vi "GetSweepData.vi"(8 "error in (no error)":errorcluster, 10 "Current Channel":string, 11 "map":T1) -> (0 "error out":errorcluster, 3 "DataSet":T2)   [LabVIEW 2017, in "EmsaTestPanel.lvlib"]
uses:
  <vilib>/addons/InsightCM/Devices/Shared/Emsa/EmsaTestPanel/EmsaTestPanel.lvlib
  <vilib>/addons/InsightCM/MessageBus/Base/controls/DataSetByteData.ctl
  <vilib>/addons/InsightCM/MessageBus/Base/controls/KeyValuePair.ctl
  <vilib>/addons/PointValueMap/controls/PointMap.ctl
  <vilib>/addons/InsightCM/Utilities/PropertyHelpers/PropertyHelpers.lvlib
  <vilib>/addons/InsightCM/Devices/Shared/Emsa/EmsaAcquisition/EmsaAcquisition.lvlib
  <vilib>/addons/InsightCM/Devices/Shared/Emsa/EmsaDataEventCreator/EmsaDataEventCreator.lvlib
  <vilib>/addons/PointValueMap/PointValueMap.lvlib
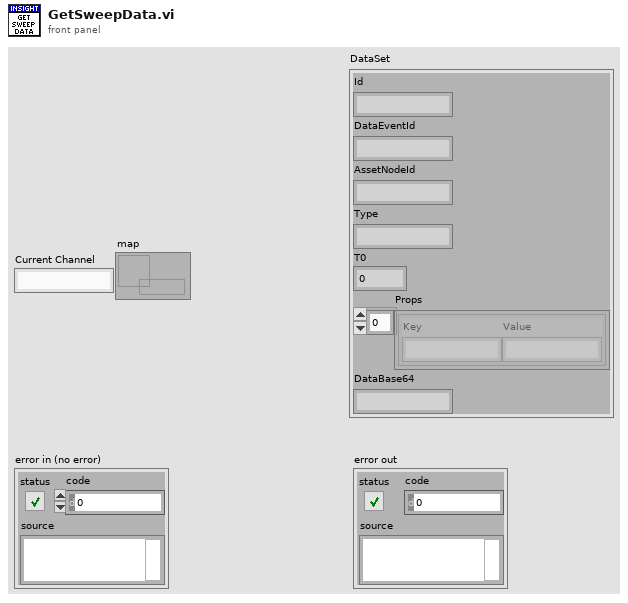
[diagram p1: front panel]
types:
  T1 = typedef "PointValueMap.lvlib/PointMap.ctl" = refnum<data-value>
  T2 = typedef "DataSetByteData.ctl" = cluster{"Id":string, "DataEventId":string, "AssetNodeId":string, "Type":string, "T0":i64, "Props":T3[], "DataBase64":string}
  T3 = typedef "KeyValuePair.ctl" = cluster{"Key":string, "Value":string}
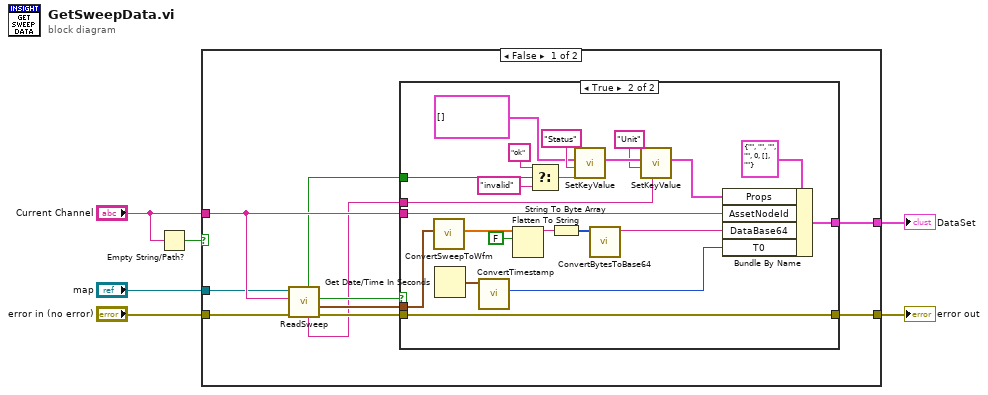
[diagram p0: block diagram]
diagram:
  n1 = Empty String/Path?(string/path="Current Channel") -> (empty?=w5:bool)
  n2 = case shown="False" w5 {
    tunnel: [w16 w40] -> w3
    tunnel: "error in (no error)" -> [w12 w40]
    tunnel: "Current Channel" -> [w14 _]
    tunnel: [w15 _] -> w2
    tunnel: "map" -> [w9 _]
    frame False {
      n3 = call <vilib>:"ReadSweep.vi"("error in (no error)"=w12, "channel"=w14, "map"=w9) -> ("error out"=w11:errorcluster, "sweep"=w10:cluster{"frequency":dbl, "amplitude":dbl}[], "found"=w13:bool, "unit"=w7:string, "valid"=w8:bool)  [unwired: 3 in, 1 out]
      n4 = case shown="True" w13 {
        tunnel: [w17 w35] -> w16
        tunnel: w11 -> [w17 w35]
        tunnel: w10 -> [_ w34]
        tunnel: w14 -> [_ w39]
        tunnel: [_ w37] -> w15
        tunnel: w8 -> [_ w30]
        tunnel: w7 -> [_ w18]
        frame False {
        }
        frame True {
          n5 = call <vilib>:"ConvertSweepToWfm.vi"("sweep"=w34) -> ("array"=w24:sgl[])  [unwired: 10 in]
          n6 = Get Date/Time In Seconds() -> (seconds since 1Jan1904=w33:timestamp)
          n7 = call <vilib>:"ConvertTimestamp.vi"("Time Stamp"=w33) -> ("Timestamp out"=w36:i64)  [unwired: 10 in]
          n8 = Flatten To String(anything=w24, prepend array or string size? (T)=FALSE) -> (data string=w25:string)  [unwired: 2 in, 2 out]
          n9 = Select(t="ok" ("hw status"), s=w30, f="invalid") -> (s? t:f=w29:string)
          n10 = String To Byte Array(string=w25) -> (unsigned byte array=w27:u8[])
          n11 = call <vilib>:"SetKeyValue.vi"("value"=w29, "key"="Status", "key value pairs"=T3[] []) -> ("key value pairs out"=w21:T3[])  [unwired: 8 in]
          n12 = call <vilib>:"ConvertBytesToBase64.vi"("U8 array"=w27) -> ("base64 encoded"=w23:string)  [unwired: 10 in]
          n13 = call <vilib>:"SetKeyValue.vi"("value"=w18, "key"="Unit", "key value pairs"=w21) -> ("key value pairs out"=w20:T3[])  [unwired: 8 in]
          n14 = Bundle By Name(cluster=T2 {"Id"="", "DataEventId"="", "AssetNodeId"="", "Type"="", "T0"=0, "Props"=[], "DataBase64"=""} ("DataSet"), "Props"=w20, "AssetNodeId"=w39, "DataBase64"=w23, "T0"=w36) -> (w37:T2)
        }
      }
    }
    frame True {
    }
  }
  "error out" <- w3
  "DataSet" <- w2
